vi "Transfer Max Bin Amplitudes.vi"   [LabVIEW 2014]
uses:
  <vilib>/rvi/Emulation/niFpgaEmulationIsFPGAContextNoSignature.vi
  <vilib>/rvi/DataTransferAndStorage/Container/Common/niFpgaContainerGetUniqueNameForEmu.vi
  <vilib>/rvi/Memory/Memory_Emulation/niFpgaMemoryEmulationCacheClearOnFirstRun.vi
  <vilib>/rvi/Memory/Memory_Emulation/nirvimemoryEmulationManagerCache_MakeExclusive.vi
  <vilib>/rvi/Memory/Memory_Emulation/niFpgaMemoryEmulationValidateCache.vi
  <vilib>/rvi/Memory/Memory_Emulation/nirvimemoryEmulationManagerCache_InsertValue.vi
  <vilib>/Utility/error.llb/Clear Errors.vi
  <vilib>/rvi/Memory/Memory_Emulation/nirvimemoryEmulationManagerCache_ReleaseExclusive.vi
  <vilib>/rvi/Memory/Memory_Emulation/nirvimemoryEmulationManagerCache_GetValue.vi
  <vilib>/rvi/Memory/Memory_Emulation/nirvimemoryEmulationManagerCache_SetValue.vi
  <vilib>/rvi/Emulation/niFpgaProcessEmulError.vi
  <vilib>/rvi/Emulation/niFpgaSctlEmulationGetInTimedLoop.vi
  <vilib>/rvi/interface/RandomDataEmulation/niFpgaRandomDataHandleErrors.vi
  <vilib>/rvi/DataTransferAndStorage/Container/XNode/niFpgaContainer.xnode
  <vilib>/rvi/DataTransferAndStorage/Register/Emulation/niFpgaRegisterEmulation.vi
  <vilib>/rvi/interface/RandomDataEmulation/nirviRandomDataFpgaReadWriteTemplate.vi
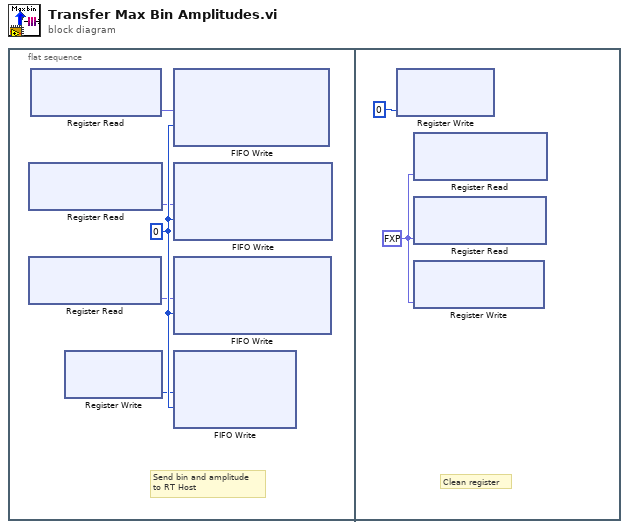
[diagram p0: block diagram]
diagram:
  n1 = flat-sequence {
    frame #0 {
      w5 = 0 ("Timeout")
      # "Send bin and amplitude\nto RT Host"
      n2 = xnode "Register Read"() -> ("Data"=w2:fxp<+,44,44>)  [unwired: 1 in, 1 out]
      n3 = xnode "Register Read"() -> ("Data"=w1:fxp<+,44,44>)  [unwired: 1 in, 1 out]
      n4 = xnode "Register Read"() -> ("Data"=w3:fxp<+,44,44>)  [unwired: 1 in, 1 out]
      n5 = xnode "Register Write"() -> ("Data"=w4:i32)  [unwired: 1 in, 1 out]
      n6 = xnode "FIFO Write"("Element"=w3, "Timeout"=w5) -> ()  [unwired: 1 in, 2 out]
      n7 = xnode "FIFO Write"("Element"=w2, "Timeout"=w5) -> ()  [unwired: 1 in, 2 out]
      n8 = xnode "FIFO Write"("Element"=w1, "Timeout"=w5) -> ()  [unwired: 1 in, 2 out]
      n9 = xnode "FIFO Write"("Element"=w4, "Timeout"=w5) -> ()  [unwired: 1 in, 2 out]
    }
    frame #1 {
      w6 = fxp<+,44,44> 0.0 ("Data")
      # "Clean register"
      n10 = xnode "Register Write"("Data"=0) -> ()  [unwired: 1 in, 1 out]
      n11 = xnode "Register Read"("Data"=w6) -> ()  [unwired: 1 in, 1 out]
      n12 = xnode "Register Read"("Data"=w6) -> ()  [unwired: 1 in, 1 out]
      n13 = xnode "Register Write"("Data"=w6) -> ()  [unwired: 1 in, 1 out]
    }
  }
